vi "Meter Detection Global Variable.vi"() -> ()   [LabVIEW 2011, in "Meter Detection Custom Device.lvlib"]
uses:
  Meter Detection Custom Device.lvlib
panel:
  in  "Needle Configuration":string="Needle Configuration"
  in  "Current Time GUID":string="8acdcb93-8529-42b6-92bf-d443b1dd904b"
  in  "Execution Time GUID":string="66ed530f-2669-461e-b2f5-508ee9997e74"
  in  "Meter Value GUID":string="25dc664e-5f40-4994-9a12-523fe15305a2"
  in  "Custom Device GUID":string="8abc71e6-051e-4bd8-bbb5-f60492892749"
  in  "Current Time":string="Current Time"
  in  "Min ROI Overlay":string="Min ROI Overlay"
  in  "Max ROI Overlay":string="Max ROI Overlay"
  in  "Points Arc":string="Points Arc"
  in  "Needle Base":string="Needle Base"
  in  "Max Meter Value":string="Max Meter Value"
  in  "Min Meter Value":string="Min Meter Value"
  in  "Camera":string="Camera"
  in  "Image":string="Image"
  in  "Max Meter ROI":string="Max Meter ROI"
  in  "Min Meter ROI":string="Min Meter ROI"
  in  "Execution Time":string="Execution Time"
  in  "Meter Value":string="Meter Value"
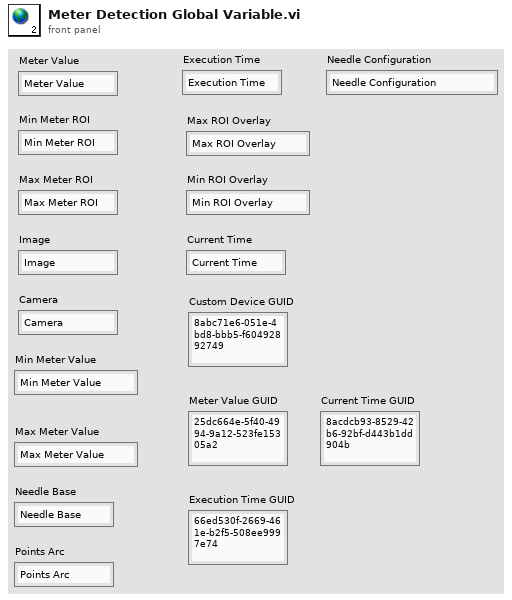
[diagram p1: front panel]
diagram:
